vi "Write File.vi"(7 "Address":string, 8 "Error In":errorcluster) -> (0 "Error Out":errorcluster)   [LabVIEW 2017, in "Tests.lvlib" / "KnownHosts.lvlib"]
uses:
  KnownHosts.lvlib
  <vilib>/Utility/error.llb/Clear Errors.vi
  <vilib>/Utility/file.llb/Is Path and Not Empty.vi
  <vilib>/Utility/sysdir.llb/Get System Directory.vi
  <vilib>/addons/_JKI Toolkits/Caraya/classes/Test/Test.lvclass
  <vilib>/addons/_JKI Toolkits/Caraya/classes/Assert/Assert.lvclass
  src/Toolkit/API/KnownHosts/KnownHosts.lvclass
  Tests.lvlib
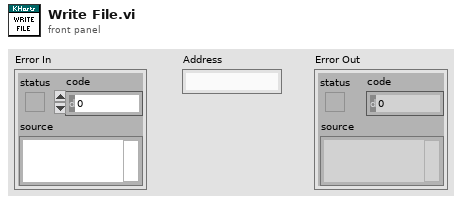
[diagram p1: front panel]
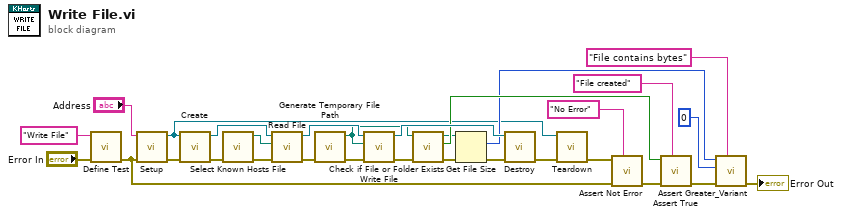
[diagram p0: block diagram]
diagram:
  n1 = call <vilib>:"Define Test.vi"("error in (no error)"="Error In", "Label (VI Title)"="Write File") -> ("error out"=w5:errorcluster)  [unwired: 9 in]
  n2 = call "Setup.vi"("Error In"=w5, "Address In"="Address") -> ("Error Out"=w4:errorcluster, "Sesssion"=w1:refnum<class "Session.lvclass">)  [unwired: 7 in, 1 out]
  n3 = call "Create.vi"("Error In"=w4, "Session"=w1) -> ("Error Out"=w26:errorcluster, "Known Hosts"=w27:refnum<class "KnownHosts.lvclass">)  [unwired: 8 in]
  n4 = call "Select Known Hosts File.vi"("Error In"=w26) -> ("Error Out"=w25:errorcluster, "Known Hosts File"=w24:path)  [unwired: 9 in]
  n5 = call "Read File.vi"("Error In"=w25, "File"=w24, "KnownHosts In"=w27) -> ("Error Out"=w21:errorcluster, "KnownHosts Out"=w23:refnum<class "KnownHosts.lvclass">)  [unwired: 6 in, 1 out]
  n6 = call <vilib>:"Generate Temporary File Path.vi"("error in (no error)"=w21) -> ("error out"=w20:errorcluster, "Unique Temporary File Path"=w18:path)  [unwired: 9 in]
  n7 = call "Write File.vi"("Error In"=w20, "File"=w18, "KnownHosts In"=w23) -> ("Error Out"=w19:errorcluster, "KnownHosts Out"=w22:refnum<class "KnownHosts.lvclass">)  [unwired: 7 in]
  n8 = call <vilib>:"Check if File or Folder Exists.vi"("error in (no error)"=w19, "path"=w18) -> ("error out"=w12:errorcluster, "file or folder exists?"=w17:bool, "dup path"=w13:path)  [unwired: 7 in]
  n9 = Get File Size(file=w13, error in=w12) -> (size (in bytes)=w8:i64, 0:w11:errorcluster)  [unwired: 1 out]
  n10 = call "Destroy.vi"("Error In"=w11, "KnownHosts"=w22) -> ("Error Out"=w3:errorcluster)  [unwired: 8 in, 1 out]
  n11 = call "Teardown.vi"("Error In"=w3, "Session"=w1) -> ("Error Out"=w2:errorcluster)  [unwired: 9 in]
  n12 = call <vilib>:"Assert Not Error.vi"("Label"="No Error", "error in (no error)"=w5, "Not Error?"=w2) -> ("error out"=w16:errorcluster)  [unwired: 8 in]
  n13 = call <vilib>:"Assert True.vi"("Label"="File created", "error in (no error)"=w16, "True?"=w17) -> ("error out"=w15:errorcluster)  [unwired: 8 in]
  n14 = call <vilib>:"Assert Greater_Variant.vi"("Label"="File contains bytes", "error in (no error)"=w15, "Y"=i64 0 ("size (in bytes)"), "X"=w8) -> ("error out"=→"Error Out":errorcluster)  [unwired: 7 in]
